vi "Main.VI"   [LabVIEW 2024]
uses:
  SUBVIS/Printer/Domino LM.lvlib
  SUBVIS/CAM/RSeries_CAM.lvlib
types:
  T1 = typedef "All Message Queues.ctl" = cluster{"DB":refnum<queue>, "Printer":refnum<queue>, "Camera":refnum<queue>, "Printer Interface":refnum<queue>, "WO":refnum<queue>}
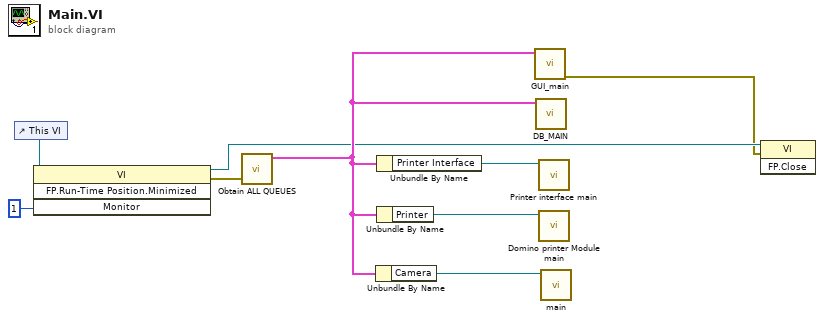
[diagram p0: block diagram]
diagram:
  n1 = control-ref of="This VI"() -> (w5:refnum<vi>)
  n2 = invoke class="VI" method="FP.Run-Time Position.Minimized"(reference=w5, "Monitor"=i16 1) -> (reference out=w3:refnum<vi>, error out=w4:errorcluster)  [unwired: 2 in, 2 out]
  n3 = call "Obtain ALL QUEUES.vi"("error in (no error)"=w4) -> ("Queues"=w6:T1)  [unwired: 9 in, 1 out]
  n4 = Unbundle By Name(w6) -> ("Camera"=w7:refnum<queue>)
  n5 = Unbundle By Name(w6) -> ("Printer Interface"=w8:refnum<queue>)
  n6 = Unbundle By Name(w6) -> ("Printer"=w9:refnum<queue>)
  n7 = call "GUI_main.vi"("Message Queues"=w6) -> ("error out"=w2:errorcluster)  [unwired: 10 in]
  n8 = call "DB_MAIN.vi"("Message Queues"=w6) -> ()  [unwired: 11 in]
  n9 = call "Printer interface main.vi"("Printer Interface"=w8) -> ()  [unwired: 11 in]
  n10 = call "Domino printer Module main.vi"("Printer"=w9) -> ()  [unwired: 11 in]
  n11 = call "main.vi"("Camera"=w7) -> ()  [unwired: 11 in]
  n12 = invoke class="VI" method="FP.Close"(reference=w3, error in=w2) -> ()  [unwired: 1 in, 3 out]
